vi "003 abreujatures 2.vi"() -> ()   [LabVIEW 2019]
panel:
  out "result string":string
  in  "stop":bool
  out "String mod":string
  in  "String":string
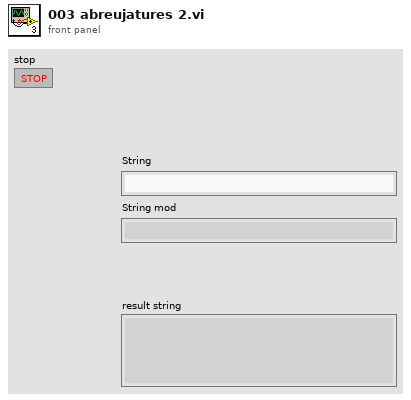
[diagram p1: front panel]
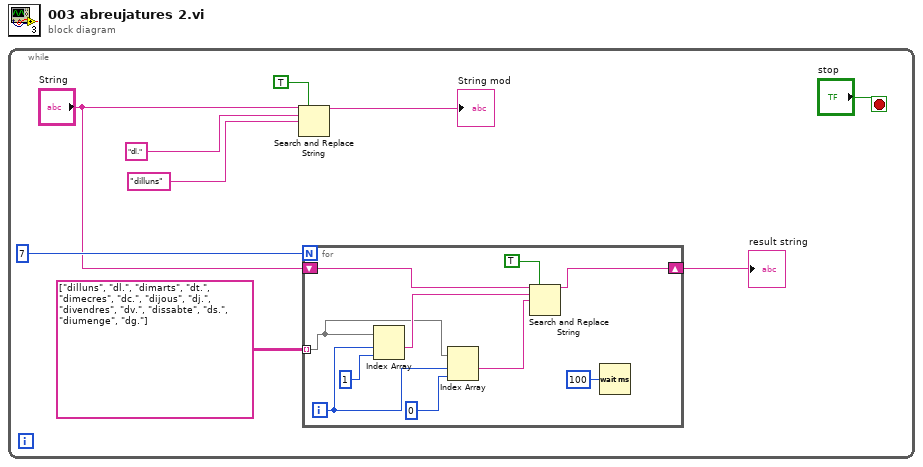
[diagram p0: block diagram]
diagram:
  n1 = while {
    stop <- "stop" stop-if-true
    n2 = Search and Replace String(replace all?=TRUE ("replace all? (F)"), input string="String", search string="dl.", replace string="dilluns" ("replace string (\"\")")) -> (result string=→"String mod":string)  [unwired: 4 in, 3 out]
    n3 = for {
      N: 7 -> [_]
      tunnel: string[][] [["dilluns", "dl."], ["dimarts", "dt."], ["dimecres", "dc."], ["dijous", "dj."], ["divendres", "dv."], ["dissabte", "ds."], ["diumenge", "dg."]] -> [w13] mode=indexing
      shift-right: [w11] -> w1
      shift-left: "String" -> [w14]
      i -> [w16]
      n4 = Index Array(array=w13, index #1=w16, index #2=1 ("index")) -> (element #1=w19:string)  [unwired: 1 out]
      n5 = Index Array(array=w13, index #1=w16, index #2=0 ("index")) -> (element #1=w15:string)  [unwired: 1 out]
      n6 = Search and Replace String(replace all?=TRUE ("replace all? (F)"), input string=w14, search string=w19, replace string=w15) -> (result string=w11:string)  [unwired: 4 in, 3 out]
      n7 = Wait (ms)(milliseconds to wait=u32 100) -> ()  [unwired: 1 out]
    }
    "result string" <- w1
  }
